vi "Polbild_ISO_pruefen.vi"(8 "Fehler in":errorcluster, 11 "Cluster in":T1={"Initialisierung"={"Online?"=FALSE, "Grundpfad"=path "", "Kamera Oben"="", "IP-Adresse Flüssiglinse"="", "Flüssiglinse"=refnum, "Kamera Unten"="", "IP-Adresse SPS"="", "SPS-Verbindung"={"TCP Connection Ref"=refnum, "IP address"="", "timeout ms"=5000, "Connected?"=FALSE, "PLC Type"=enum."S7 1200", "Rack S7 400"=0, "Slot S7 400"=0, "PDU Size"=0, "connection semaphore"=refnum}, "IP-Adresse Lichtgitter"="", "Lichtgitter"=refnum, "Skalierungsfaktor"=0.0, "Bilder Oben"=[], "Bild Unten"=refnum, "Bild Ausschnitt Unten"=refnum}, "Einstellungen"={"Gesamtablauf gestartet"=FALSE, "i. O. Bilder speichern"=FALSE, "Bildspeicherung Offline"=FALSE, "Ausgewähltes Offline-Datum"="", "Ausgewähltes Offline-Teil"="", "Speicherpfad Bilder"=path ""}, "Artikeldaten"={"Artikelnummer"="", "Fertigungsauftrag"="", "Muster ISO"=refnum, "Belichtungszeit Referenzmarken"=0.0, "Fokus Referenzmarken"=0.0, "Belichtungszeit ISO"=0.0, "Fokus ISO"=0.0, "Belichtungszeit Unten"=0.0, "Kontaktanzahl"=0, "Aktueller Kontakt"=0, "Kontaktposition"={"x"=0.0, "y"=0.0}, "Winkel ISO"=0.0, "ISO-Muster nicht vorhanden"=FALSE}, "Werte Kamera Oben"={"Koordinatensystem"={"Punkt x-Achse"={"X"=0.0, "Y"=0.0}, "Ursprung"={"X"=0.0, "Y"=0.0}, "Punkt y-Achse"={"X"=0.0, "Y"=0.0}}, "Position Kontakt"={"x"=0.0, "y"=0.0}, "Winkel Kontakt"=0.0}, "Werte Kamera Unten"={"Prüfung Unten n. i. O."=FALSE}, "Werte Lichtgitter"={"Messwerte Referenzmarken"=[], "Mittelpunkt Referenzmarken"={"x"=0.0, "y"=0.0}, "Messwerte Kontakt"=[], "Offset"={"x"=0.0, "y"=0.0}}, "Rückmeldungen"={"Koordinaten ermittelt"=FALSE, "Vermessung Lichtgitter fertig"=FALSE, "Nachkontrolle Kamera Unten fertig"=FALSE}, "Fehler"={"Referenzen nicht gefunden"=FALSE, "Kontakt nicht gefunden"=FALSE, "Referenzen nicht in Lichtgitter"=FALSE, "Kontakt zu groß"=FALSE, "Kontakt zu klein"=FALSE}, "Statistik"={"Statistiken"=[]}, "Timer"={"Timer Start Position"=0, "Timer Start Lichtgitter"=0, "Timer Start Kamera Unten"=0}}) -> (0 "Fehler out":errorcluster, 2 "Polbild i.O.":bool, 3 "Cluster out":T1={"Initialisierung"={"Online?"=FALSE, "Grundpfad"=path "", "Kamera Oben"="", "IP-Adresse Flüssiglinse"="", "Flüssiglinse"=refnum, "Kamera Unten"="", "IP-Adresse SPS"="", "SPS-Verbindung"={"TCP Connection Ref"=refnum, "IP address"="", "timeout ms"=5000, "Connected?"=FALSE, "PLC Type"=enum."S7 1200", "Rack S7 400"=0, "Slot S7 400"=0, "PDU Size"=0, "connection semaphore"=refnum}, "IP-Adresse Lichtgitter"="", "Lichtgitter"=refnum, "Skalierungsfaktor"=0.0, "Bilder Oben"=[], "Bild Unten"=refnum, "Bild Ausschnitt Unten"=refnum}, "Einstellungen"={"Gesamtablauf gestartet"=FALSE, "i. O. Bilder speichern"=FALSE, "Bildspeicherung Offline"=FALSE, "Ausgewähltes Offline-Datum"="", "Ausgewähltes Offline-Teil"="", "Speicherpfad Bilder"=path ""}, "Artikeldaten"={"Artikelnummer"="", "Fertigungsauftrag"="", "Muster ISO"=refnum, "Belichtungszeit Referenzmarken"=0.0, "Fokus Referenzmarken"=0.0, "Belichtungszeit ISO"=0.0, "Fokus ISO"=0.0, "Belichtungszeit Unten"=0.0, "Kontaktanzahl"=0, "Aktueller Kontakt"=0, "Kontaktposition"={"x"=0.0, "y"=0.0}, "Winkel ISO"=0.0, "ISO-Muster nicht vorhanden"=FALSE}, "Werte Kamera Oben"={"Koordinatensystem"={"Punkt x-Achse"={"X"=0.0, "Y"=0.0}, "Ursprung"={"X"=0.0, "Y"=0.0}, "Punkt y-Achse"={"X"=0.0, "Y"=0.0}}, "Position Kontakt"={"x"=0.0, "y"=0.0}, "Winkel Kontakt"=0.0}, "Werte Kamera Unten"={"Prüfung Unten n. i. O."=FALSE}, "Werte Lichtgitter"={"Messwerte Referenzmarken"=[], "Mittelpunkt Referenzmarken"={"x"=0.0, "y"=0.0}, "Messwerte Kontakt"=[], "Offset"={"x"=0.0, "y"=0.0}}, "Rückmeldungen"={"Koordinaten ermittelt"=FALSE, "Vermessung Lichtgitter fertig"=FALSE, "Nachkontrolle Kamera Unten fertig"=FALSE}, "Fehler"={"Referenzen nicht gefunden"=FALSE, "Kontakt nicht gefunden"=FALSE, "Referenzen nicht in Lichtgitter"=FALSE, "Kontakt zu groß"=FALSE, "Kontakt zu klein"=FALSE}, "Statistik"={"Statistiken"=[]}, "Timer"={"Timer Start Position"=0, "Timer Start Lichtgitter"=0, "Timer Start Kamera Unten"=0}})   [LabVIEW 2024]
uses:
  Cluster.ctl
  Kontaktmontagemodul.exe/1abvi3w/vi.lib/userDefined/High Color/IMAQdx.ctl
  Kontaktmontagemodul.exe/1abvi3w/vi.lib/DATA AHEAD/SP7/typedefs/S7 Connection.ctl
  Kontaktmontagemodul.exe/1abvi3w/vi.lib/DATA AHEAD/SP7/typedefs/PLC Type.ctl
  Kontaktmontagemodul.exe/1abvi3w/vi.lib/vision/Image Controls.llb/IMAQ Image.ctl
  Koordinatensystem.ctl
  Statistik.ctl
  Kontaktmontagemodul.exe/1abvi3w/vi.lib/vision/NI_Vision_Development_Module.lvlib
  Kontaktmontagemodul.exe/1abvi3w/vi.lib/DATA AHEAD/SP7/SP7.lvlib
panel:
  out "Number of Matches":i32
  out "Zeit Pattern Matching":u32
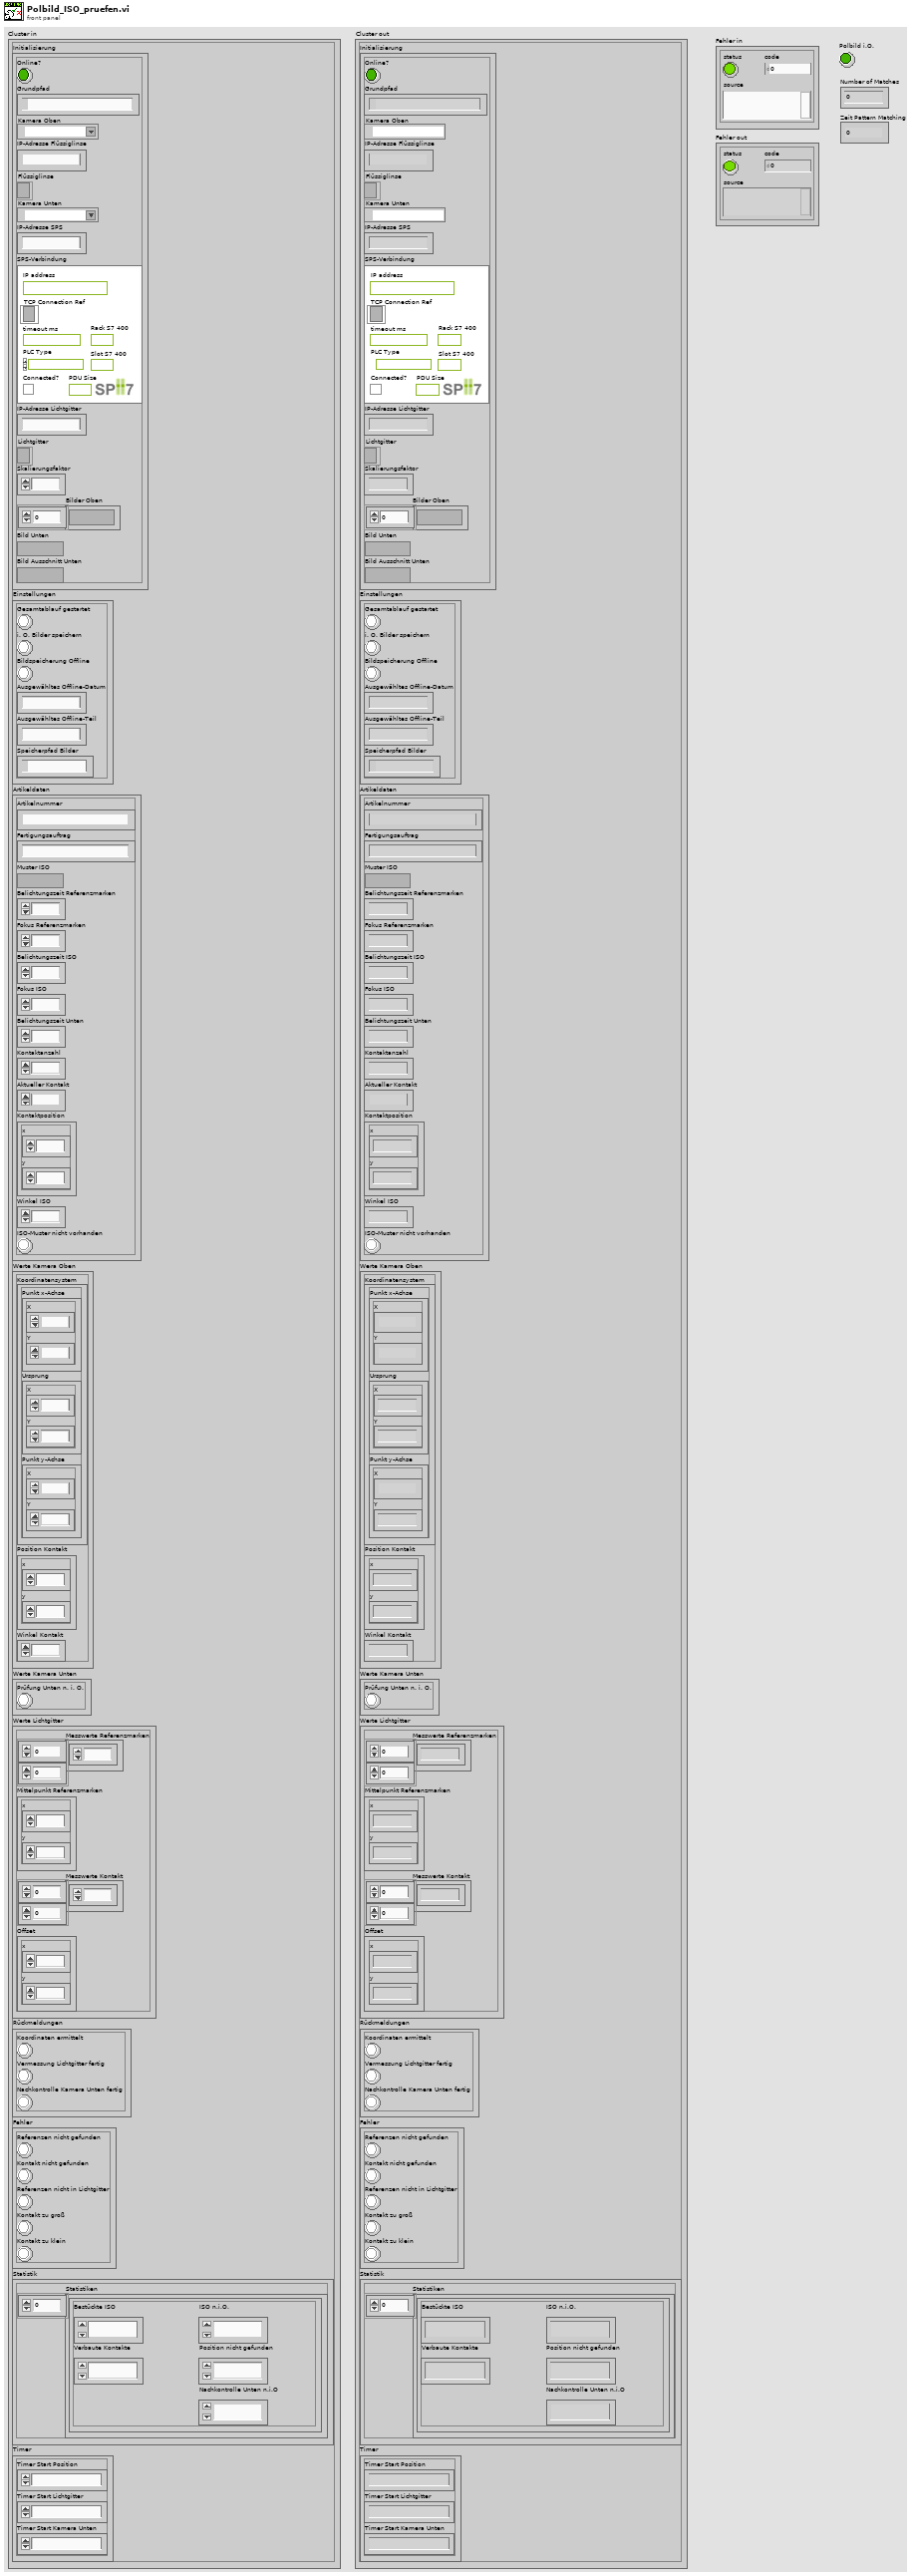
[diagram p1: front panel]
types:
  T1 = typedef "Cluster.ctl" = cluster{"Initialisierung":cluster{"Online?":bool, "Grundpfad":path, "Kamera Oben":T2, "IP-Adresse Flüssiglinse":string, "Flüssiglinse":refnum<k5>, "Kamera Unten":T2, "IP-Adresse SPS":string, "SPS-Verbindung":T3, "IP-Adresse Lichtgitter":string, "Lichtgitter":refnum<k5>, "Skalierungsfaktor":dbl, "Bilder Oben":T6[], "Bild Unten":T6, "Bild Ausschnitt Unten":T6}, "Einstellungen":cluster{"Gesamtablauf gestartet":bool, "i. O. Bilder speichern":bool, "Bildspeicherung Offline":bool, "Ausgewähltes Offline-Datum":string, "Ausgewähltes Offline-Teil":string, "Speicherpfad Bilder":path}, "Artikeldaten":cluster{"Artikelnummer":string, "Fertigungsauftrag":string, "Muster ISO":T6, "Belichtungszeit Referenzmarken":dbl, "Fokus Referenzmarken":dbl, "Belichtungszeit ISO":dbl, "Fokus ISO":dbl, "Belichtungszeit Unten":dbl, "Kontaktanzahl":u32, "Aktueller Kontakt":i16, "Kontaktposition":cluster{"x":sgl, "y":sgl}, "Winkel ISO":sgl, "ISO-Muster nicht vorhanden":bool}, "Werte Kamera Oben":cluster{"Koordinatensystem":T7, "Position Kontakt":cluster{"x":dbl, "y":dbl}, "Winkel Kontakt":dbl}, "Werte Kamera Unten":cluster{"Prüfung Unten n. i. O.":bool}, "Werte Lichtgitter":cluster{"Messwerte Referenzmarken":dbl[][], "Mittelpunkt Referenzmarken":cluster{"x":dbl, "y":dbl}, "Messwerte Kontakt":dbl[][], "Offset":cluster{"x":dbl, "y":dbl}}, "Rückmeldungen":cluster{"Koordinaten ermittelt":bool, "Vermessung Lichtgitter fertig":bool, "Nachkontrolle Kamera Unten fertig":bool}, "Fehler":cluster{"Referenzen nicht gefunden":bool, "Kontakt nicht gefunden":bool, "Referenzen nicht in Lichtgitter":bool, "Kontakt zu groß":bool, "Kontakt zu klein":bool}, "Statistik":cluster{"Statistiken":T8[]}, "Timer":cluster{"Timer Start Position":u32, "Timer Start Lichtgitter":u32, "Timer Start Kamera Unten":u32}}
  T2 = typedef "IMAQdx.ctl" = refnum<k21>
  T3 = typedef "SP7.lvlib/S7 Connection.ctl" = cluster{"TCP Connection Ref":refnum<k5>, "IP address":string, "timeout ms":i32, "Connected?":bool, "PLC Type":T4, "Rack S7 400":u8, "Slot S7 400":u8, "PDU Size":u16, "connection semaphore":T5}
  T4 = typedef "SP7.lvlib/PLC Type.ctl" = enum16{"S7 200", "S7 300/400", "S7 1200", "S7 1500", "LOGO!8"}
  T5 = typedef "Semaphore RefNum" = refnum<k1>
  T6 = typedef "IMAQ Image.ctl" = refnum<image>
  T7 = typedef "Koordinatensystem.ctl" = cluster{"Punkt x-Achse":cluster{"X":sgl, "Y":sgl}, "Ursprung":cluster{"X":sgl, "Y":sgl}, "Punkt y-Achse":cluster{"X":sgl, "Y":sgl}}
  T8 = typedef "Statistik.ctl" = cluster{"Bestückte ISO":u32, "Verbaute Kontakte":u32, "ISO n.i.O.":u32, "Nachkontrolle Unten n.i.O":u32, "Position nicht gefunden":u32}
  T9 = cluster{"Number of Matches Requested":i32, "Minimum Match Score":sgl, "Angle Ranges":cluster{"Start Angle":sgl, "End Angle":sgl}[]}
  T10 = cluster{"Position":cluster{"x":sgl, "y":sgl}, "Angle":sgl, "Scale":sgl, "Score":sgl, "Bounding Box":cluster{"x":sgl, "y":sgl}[]}[]
  T11 = cluster{"Position":cluster{"x":sgl, "y":sgl}, "Angle":sgl, "Scale":sgl, "Score":sgl, "Bounding Box":cluster{"x":sgl, "y":sgl}[]}
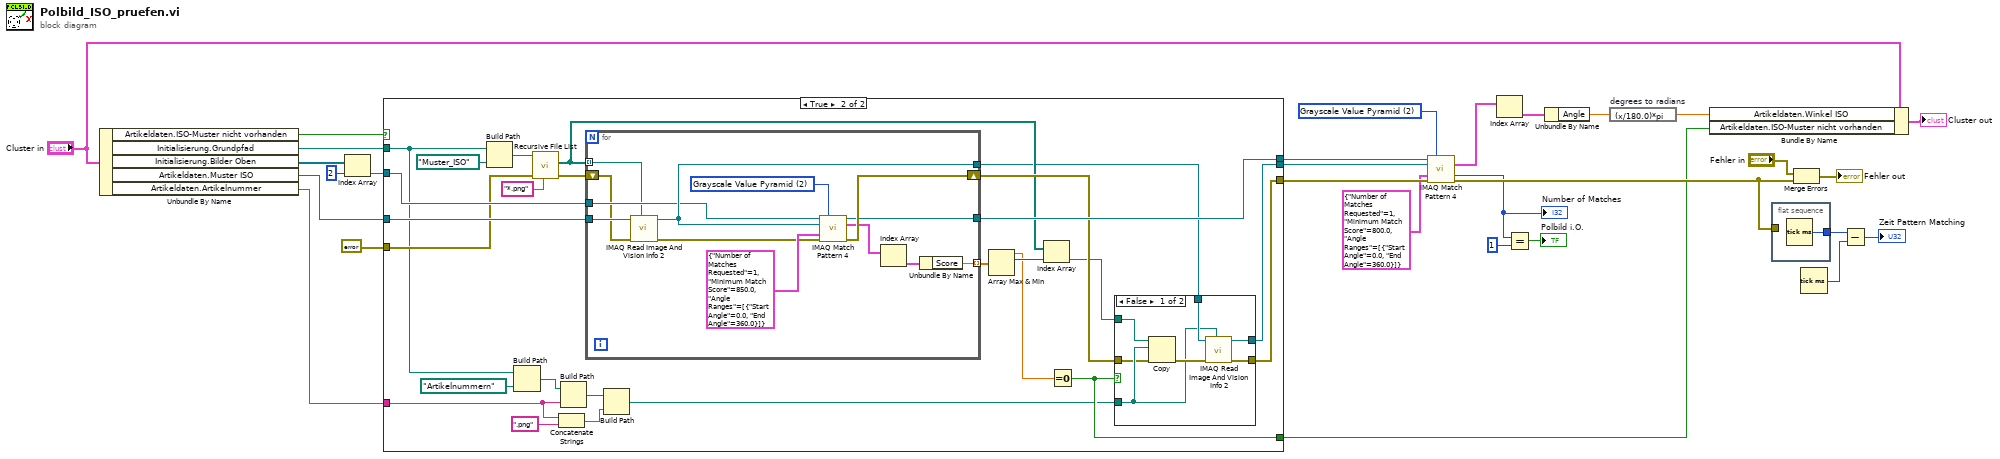
[diagram p0: block diagram]
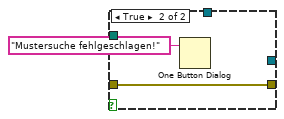
[diagram p3: hidden frame]
diagram:
  w2 = 2 items=["All", "Low Discrepancy Sampling", "Grayscale Value Pyramid", "Gradients Pyramid"] ("Algorithm")
  n1 = Unbundle By Name("Cluster in") -> ("Artikeldaten.ISO-Muster nicht vorhanden"=w17:bool, "Initialisierung.Grundpfad"=w16:path, "Initialisierung.Bilder Oben"=w15:T6[], "Artikeldaten.Muster ISO"=w13:T6, "Artikeldaten.Artikelnummer"=w11:string)
  n2 = Index Array(array=w15, index=2) -> (element=w14:T6)
  n3 = case shown="True" w17 {
    tunnel: w16 -> [_ w50]
    tunnel: [w30 w43] -> w4
    tunnel: w13 -> [w31 w55]
    tunnel: [w31 w38] -> w5
    tunnel: w14 -> [w32 w54]
    tunnel: errorcluster {"status"=FALSE, "code"=0, "source"=""} ("error in") -> [w30 w52]
    tunnel: [w32 w51] -> w12
    tunnel: w11 -> [_ w36]
    tunnel: [_ w40] -> w8
    frame False {
    }
    frame True {
      n4 = Build Path(base path=w50, name or relative path=path "Muster_ISO") -> (appended path=w57:path)
      n5 = Build Path(base path=w50, name or relative path=path "Artikelnummern") -> (appended path=w48:path)
      n6 = call "Recursive File List.vi"("pattern"="*.png", "error in (no error)"=w52, "Folder Path"=w57) -> ("error out"=w53:errorcluster, "All Files in Dir"=w44:path[])  [unwired: 4 in, 3 out]
      n7 = Concatenate Strings(w36, ".png" ("string")) -> (w34:string)
      n8 = Build Path(base path=w48, name or relative path=w36) -> (appended path=w35:path)
      n9 = for {
        tunnel: w44 -> [w62] mode=indexing
        tunnel: w55 -> [w69]
        tunnel: [w68] -> w39
        tunnel: w54 -> [w67]
        shift-right: [w64] -> w47
        shift-left: w53 -> [w66]
        tunnel: [w63] -> w51
        tunnel: [w59] -> w46 mode=indexing
        w70 = 2 items=["All", "Low Discrepancy Sampling", "Grayscale Value Pyramid", "Gradients Pyramid"] ("Algorithm")
        n10 = call "IMAQ Read Image And Vision Info 2"("File Path"=w62, "error in (no error)"=w66, "Image"=w69) -> ("error out"=w65:errorcluster, "Image Out"=w68:T6)  [unwired: 6 in, 1 out]
        n11 = call "IMAQ Match Pattern 4"("Image"=w67, "Algorithm"=w70, "Template Image"=w68, "Parameters"=T9 {"Number of Matches Requested"=1, "Minimum Match Score"=850.0, "Angle Ranges"=[{"Start Angle"=0.0, "End Angle"=360.0}]}, "error in (no error)"=w65) -> ("Image (duplicate)"=w63:T6, "Matches (pixel)"=w61:T10, "error out"=w64:errorcluster)  [unwired: 6 in, 2 out]
        n12 = Index Array(array=w61) -> (element=w60:T11)  [unwired: 1 in]
        n13 = Unbundle By Name(w60) -> ("Score"=w59:sgl)
      }
      n14 = Build Path(base path=w35, name or relative path=w34) -> (appended path=w33:path)
      n15 = Array Max & Min(array=w46) -> (max value=w41:sgl, max index (indices)=w45:i32)  [unwired: 2 out]
      n16 = Index Array(array=w44, index=w45) -> (element=w42:path)
      n17 = Equal To 0?(x=w41) -> (x = 0?=w40:bool)
      n18 = case shown="False" w40 {
        tunnel: w47 -> [w72 w80]
        tunnel: [w76 w80] -> w43
        tunnel: w42 -> [w78 _]
        tunnel: w39 -> [w75 _]
        tunnel: [w74 _] -> w38
        tunnel: w33 -> [w73 _]
        frame False {
          n19 = Copy(8:w72, 10:w73, 11:w78) -> (0:w77:errorcluster)  [unwired: 2 in, 2 out]
          n20 = call "IMAQ Read Image And Vision Info 2"("File Path"=w73, "error in (no error)"=w77, "Image"=w75) -> ("error out"=w76:errorcluster, "Image Out"=w74:T6)  [unwired: 6 in, 1 out]
        }
        frame True {
          n21 = One Button Dialog(message="Mustersuche fehlgeschlagen!") -> ()  [unwired: 1 in, 1 out]
        }
      }
    }
  }
  n22 = call "IMAQ Match Pattern 4"("Image"=w12, "Algorithm"=w2, "Template Image"=w5, "Parameters"=T9 {"Number of Matches Requested"=1, "Minimum Match Score"=800.0, "Angle Ranges"=[{"Start Angle"=0.0, "End Angle"=360.0}]}, "error in (no error)"=w4) -> ("Matches (pixel)"=w22:T10, "Number of Matches"=w1:i32, "error out"=w10:errorcluster)  [unwired: 6 in, 2 out]
  "Number of Matches" <- w1
  n23 = Index Array(array=w22) -> (element=w21:T11)  [unwired: 1 in]
  n24 = Equal?(x=w1, y=1) -> (x = y?=→"Polbild i.O.":bool)
  n25 = Unbundle By Name(w21) -> ("Angle"=w24:sgl)
  n26 = expression code="(x/180.0)*pi" "degrees to radians"(w24) -> (w26:sgl)
  n27 = Bundle By Name(cluster="Cluster in", "Artikeldaten.Winkel ISO"=w26, "Artikeldaten.ISO-Muster nicht vorhanden"=w8) -> (→"Cluster out":T1)
  n28 = flat-sequence {
    tunnel: [w81] -> w20
    tunnel: w10 -> [_]
    frame #0 {
      n29 = Tick Count (ms)() -> (millisecond timer value=w81:u32)
    }
  }
  n30 = Merge Errors("Fehler in", w10) -> (→"Fehler out":errorcluster)
  n31 = Tick Count (ms)() -> (millisecond timer value=w19:u32)
  n32 = Subtract(x=w20, y=w19) -> (x-y=→"Zeit Pattern Matching":u32)
